vi "Octal Channel Open AOTF.vi"(0 "AOTF Index":i32, 11 "Error In":errorcluster) -> (4 "AOTF Handle":u64, 15 "Error Out":errorcluster)   [LabVIEW 2020]
uses:
  Program Files/Crystal Technology/Developer/AotfLibrary/Dll/AotfLibrary.dll
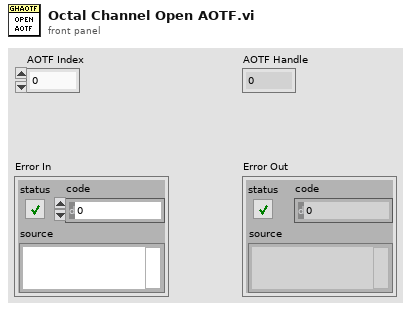
[diagram p1: front panel]
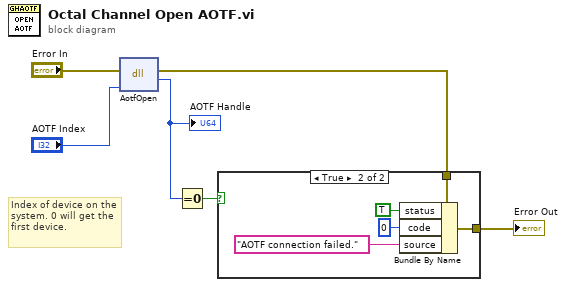
[diagram p0: block diagram]
diagram:
  # "Index of device on the system. 0 will get the first device."
  n1 = dll-call lib="C:/Program Files/Crystal Technology/Developer/AotfLibrary/Dll/AotfLibrary.dll" fn="AotfOpen"(error in="Error In", "iInstance"="AOTF Index") -> (error out=w2:errorcluster, "Handle"=w5:u64)  [unwired: 3 in, 1 out]
  "AOTF Handle" <- w5
  n2 = Equal To 0?(x=w5) -> (x = 0?=w6:bool)
  n3 = case shown="True" w6 {
    tunnel: w2 -> [w7 w9]
    tunnel: [w7 w8] -> w1
    frame False {
    }
    frame True {
      n4 = Bundle By Name(cluster=w9, "status"=TRUE, "code"=0, "source"="AOTF connection failed.") -> (w8:errorcluster)
    }
  }
  "Error Out" <- w1
